vi "find_patches_test.vi"() -> ()   [LabVIEW 2023]
uses:
  find_patches parameters.ctl
  Vision.lvlib
panel:
  out "log out":string
  in  "Field of View":cluster{"fieldOfViewX":sgl, "fieldOfViewY":sgl}={"fieldOfViewX"=1.4, "fieldOfViewY"=1.048}
  in  "find_patches parameters":T1={"dilateSize"=5, "sizeMin"=0.2, "sizeMax"=0.4, "aspectRatioMin"=0.9, "aspectRatioMax"=1.1, "colorGroups"=2}
  out "Patches":T2(array[cluster]) {"x" format="%#_3g"; "y" format="%#_3g"; "aspect ratio" format="%#_3g"; "size" format="%#_3g"; "image-x" format="%#_3g"; "image-y" format="%#_3g"}
  out "Number of Fiducials":i32
  in  "File Path":path=path "C:/Users/cfang/Desktop/pixel-gantry-control/Data/HDI_fid.png"
  out "error out":errorcluster
  out "Image":T3(plugin-control)
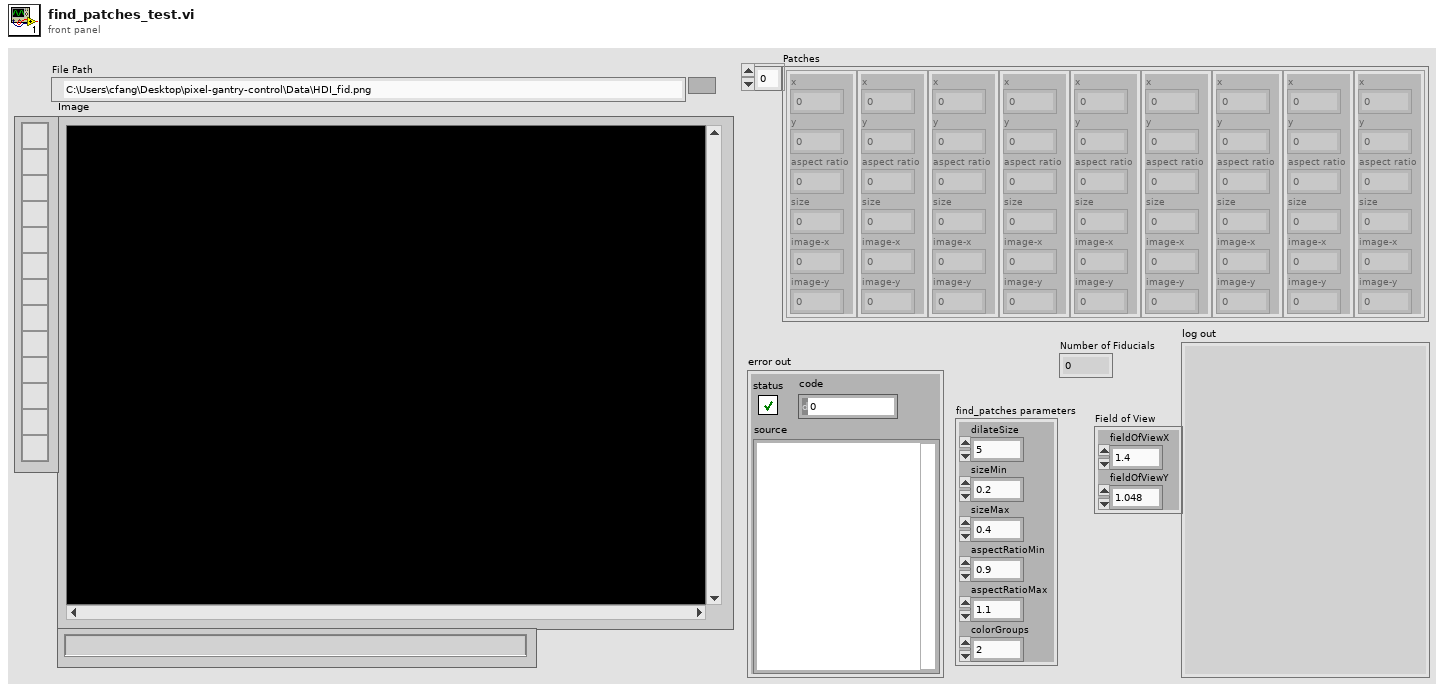
[diagram p1: front panel]
types:
  T1 = typedef "Vision.lvlib/find_patches parameters.ctl" = cluster{"dilateSize":i32, "sizeMin":sgl, "sizeMax":sgl, "aspectRatioMin":sgl, "aspectRatioMax":sgl, "colorGroups":i32}
  T2 = cluster{"x":dbl, "y":dbl, "aspect ratio":dbl, "size":dbl, "image-x":dbl, "image-y":dbl}[]
  T3 = typedef "IMAQ Image.ctl" = refnum<image>
  T4 = cluster{"Left":i32, "Top":i32, "Right":i32, "Bottom":i32}
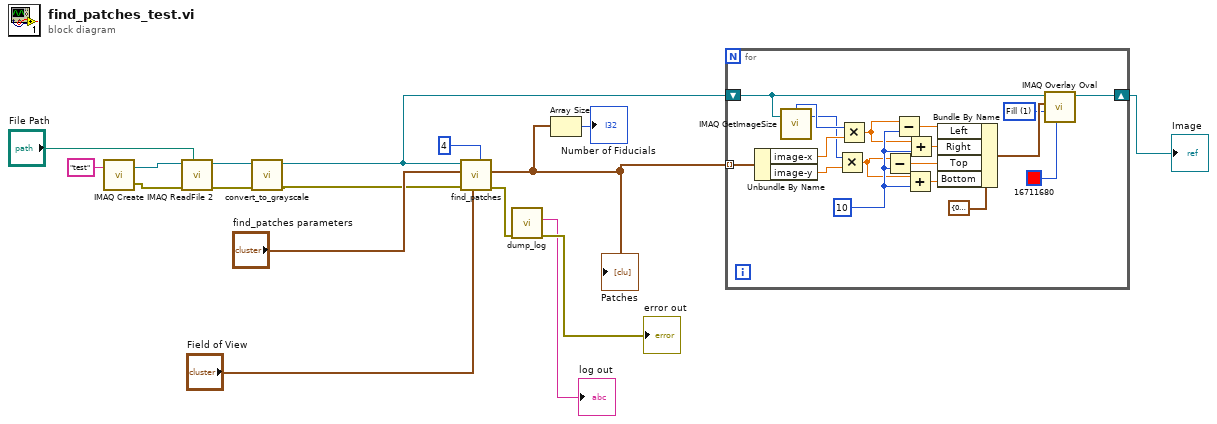
[diagram p0: block diagram]
diagram:
  n1 = call "IMAQ Create"("Image Name"="test") -> ("New Image"=w17:T3, "error out"=w15:errorcluster)  [unwired: 4 in]
  n2 = call "IMAQ ReadFile 2"("File Path"="File Path", "error in (no error)"=w15, "Image"=w17) -> ("error out"=w5:errorcluster, "Image Out"=w7:T3)  [unwired: 4 in, 3 out]
  n3 = call "convert_to_grayscale.vi"("error in (no error)"=w5, "Image in"=w7) -> ("error out"=w4:errorcluster, "Image out"=w6:T3)  [unwired: 8 in]
  n4 = call "find_patches.vi"("Shrink Factor"=4, "Field of View"="Field of View", "error in"=w4, "find_patches parameters"="find_patches parameters", "Image"=w6) -> ("error out"=w3:errorcluster, "Patches"=w9:T2)  [unwired: 5 in]
  "Patches" <- w9
  n5 = call "dump_log.vi"("error in (no error)"=w3) -> ("error out"=→"error out":errorcluster, "log out"=→"log out":string)  [unwired: 9 in]
  n6 = Array Size(array=w9) -> (size(s)=→"Number of Fiducials":i32)
  n7 = for {
    tunnel: w9 -> [w35] mode=indexing
    shift-right: [w19] -> w8
    shift-left: w6 -> [w30]
    w18 = u32 1 items=["Frame", "Fill"] ("Drawing Mode (Frame)")
    w23 = 10
    n8 = Unbundle By Name(w35) -> ("image-x"=w34:dbl, "image-y"=w32:dbl)
    n9 = call "IMAQ GetImageSize"("Image"=w30) -> ("Y Resolution"=w31:i32, "X Resolution"=w33:i32)  [unwired: 3 in, 1 out]
    n10 = Multiply(x=w31, y=w32) -> (x*y=w22:dbl)
    n11 = Multiply(x=w33, y=w34) -> (x*y=w21:dbl)
    n12 = Subtract(x=w22, y=w23) -> (x-y=w24:dbl)
    n13 = Subtract(x=w21, y=w23) -> (x-y=w25:dbl)
    n14 = Add(x=w22, y=w23) -> (x+y=w26:dbl)
    n15 = Add(x=w21, y=w23) -> (x+y=w27:dbl)
    n16 = Bundle By Name(cluster=T4 {"Left"=0, "Top"=0, "Right"=0, "Bottom"=0} ("Bounding Rectangle"), "Left"=w25, "Right"=w27, "Top"=w24, "Bottom"=w26) -> (w20:T4)
    n17 = call "IMAQ Overlay Oval"("Color"=u32 16711680, "Drawing Mode (Frame)"=w18, "Bounding Rectangle"=w20, "Image"=w30) -> ("Image Out"=w19:T3)  [unwired: 6 in, 1 out]
  }
  "Image" <- w8
